vi "Save config.vi"(8 "error in (no error)":errorcluster, 11 "Config":T1={"Arduino port"="COM4", "Starting angle M1"=0.0, "Starting angle M2"=0.0}) -> (0 "error out":errorcluster)   [LabVIEW 2020]
uses:
  <vilib>/Utility/config.llb/NI_LVConfig.lvlib
  <vilib>/Utility/config.llb/Write Key (Double).vi
  <vilib>/Utility/config.llb/Write Key (String).vi
  Controls/Config -- cluster.ctl
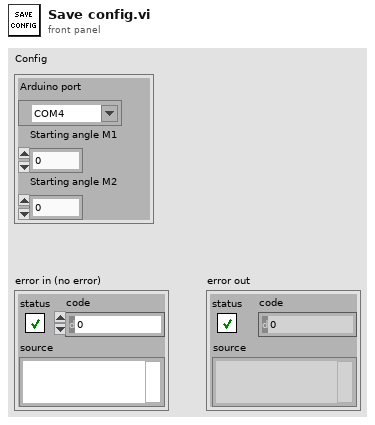
[diagram p1: front panel]
types:
  T1 = typedef "Config -- cluster.ctl" = cluster{"Arduino port":refnum<visa-resource-name>, "Starting angle M1":dbl, "Starting angle M2":dbl}
  T2 = typedef "NI_LVConfig.lvlib/Config Data RefNum.ctl" = refnum<k1>
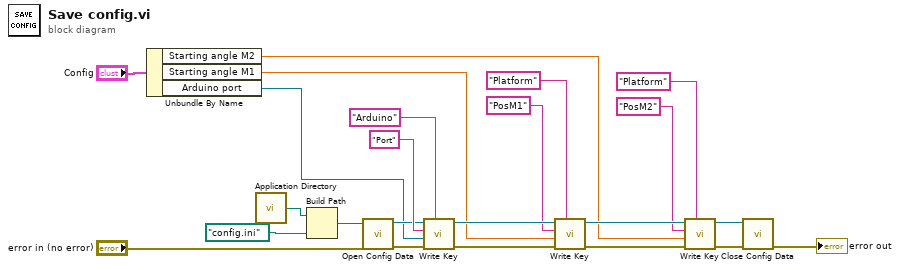
[diagram p0: block diagram]
diagram:
  n1 = Unbundle By Name("Config") -> ("Starting angle M2"=w1:dbl, "Starting angle M1"=w2:dbl, "Arduino port"=w3:refnum<visa-resource-name>)
  n2 = call <vilib>:"Application Directory.vi"() -> ("Application Directory"=w7:path)
  n3 = Build Path(base path=w7, name or relative path=path "config.ini") -> (appended path=w9:path)
  n4 = call <vilib>:"Open Config Data.vi"("error in (no error)"="error in (no error)", "configuration file path"=w9) -> ("error out"=w10:errorcluster, "refnum"=w11:T2)  [unwired: 7 in, 1 out]
  n5 = call-poly <vilib>:"Write Key.vi"("section"="Arduino", "error in (no error)"=w10, "value"=w3, "key"="Port", "refnum"=w11) -> ("error out"=w14:errorcluster, "refnum out"=w17:T2)  [unwired: 4 in, 1 out]
  n6 = call-poly <vilib>:"Write Key.vi"("section"="Platform", "error in (no error)"=w14, "value"=w2, "key"="PosM1", "refnum"=w17) -> ("error out"=w21:errorcluster, "refnum out"=w20:T2)  [unwired: 4 in, 1 out]
  n7 = call-poly <vilib>:"Write Key.vi"("section"="Platform", "error in (no error)"=w21, "value"=w1, "key"="PosM2", "refnum"=w20) -> ("error out"=w22:errorcluster, "refnum out"=w23:T2)  [unwired: 4 in, 1 out]
  n8 = call <vilib>:"Close Config Data.vi"("error in (no error)"=w22, "refnum"=w23) -> ("error out"=→"error out":errorcluster)  [unwired: 8 in, 1 out]
